vi "1A_Get User Input Start.vi"(1 "Serial Number In":string) -> (0 "fXpgIdentity Output":T1)   [LabVIEW 2010]
panel:
  in  "Stellar \"QIG\" Serial Number":string
  in  "Continue Button":bool
  in  "Device SERIAL Number":string
  in  "PCB LOT Number":string
  # "Enter All Device Parameters Below.\nWhen finished, click \"Continue\"."
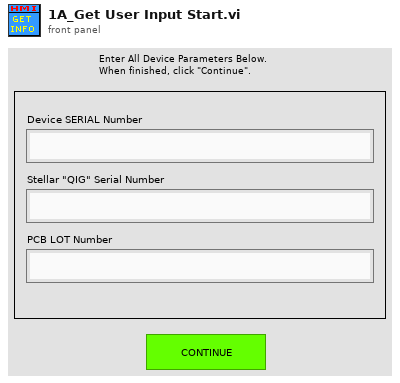
[diagram p1: front panel]
types:
  T1 = cluster{"xpgPCBLotNumber":string, "xpgSerialNumber[20]":string, "xpgStellarQIGSerialNumber":string}
  T2 = cluster{"xpgPCBLOTNumber":string, "xpgSerialNumber[20]":string, "xpgStellarQIGSerialNumber":string}
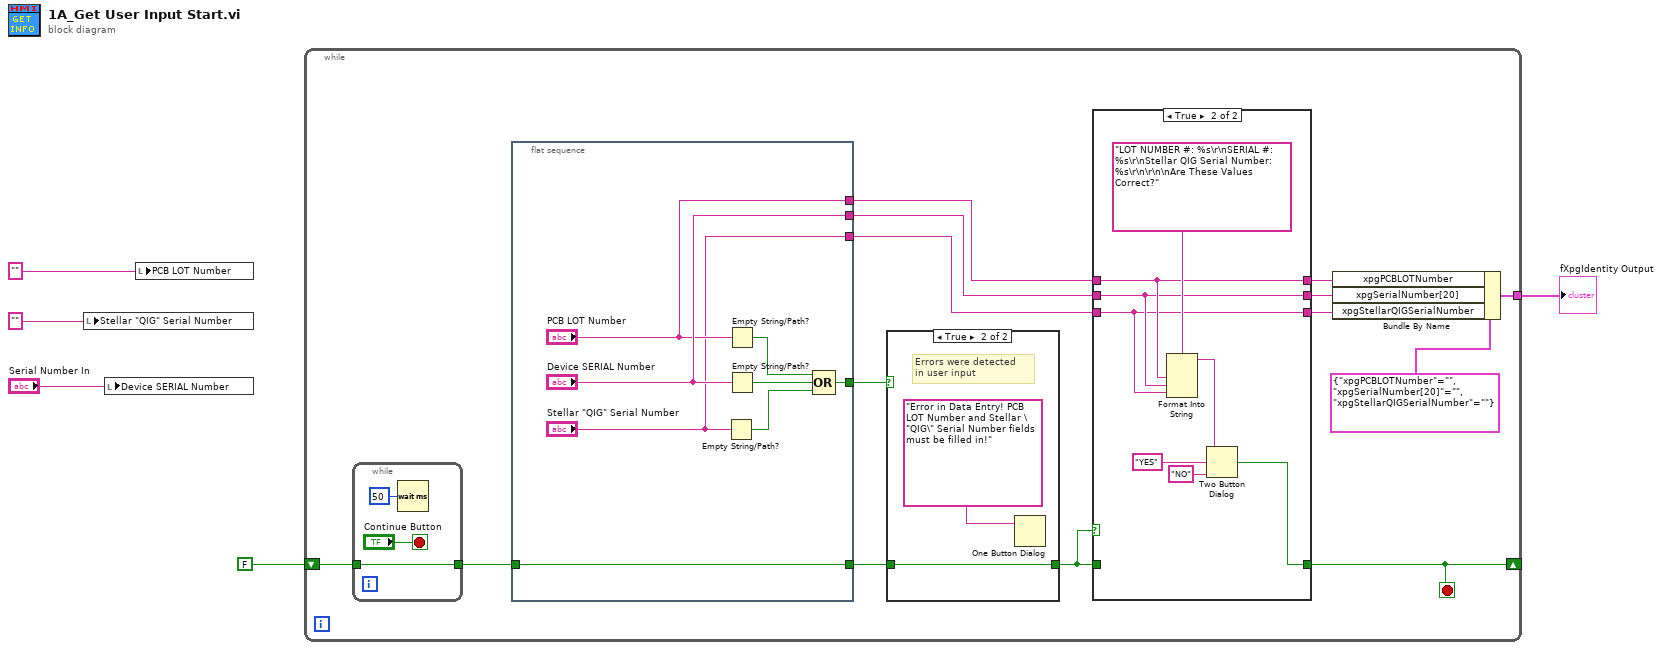
[diagram p0: block diagram]
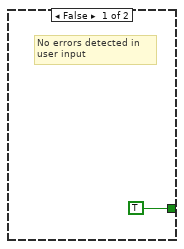
[diagram p3: hidden frame]
diagram:
  n1 = local write "Stellar \"QIG\" Serial Number"("" ("Device LOT Number")) -> ()
  n2 = local write "Device SERIAL Number"("Serial Number In") -> ()
  n3 = local write "PCB LOT Number"("" ("Device LOT Number")) -> ()
  n4 = while {
    shift-right: [w12] -> _
    shift-left: FALSE -> [w19]
    tunnel: [w10] -> w3
    stop <- w12 stop-if-true
    n5 = while {
      tunnel: w19 -> [w45]
      tunnel: [w45] -> w17
      stop <- "Continue Button" stop-if-true
      n6 = Wait (ms)(milliseconds to wait=u32 50) -> ()  [unwired: 1 out]
    }
    n7 = flat-sequence {
      tunnel: [w37] -> w18
      tunnel: ["Device SERIAL Number"] -> w13
      tunnel: ["PCB LOT Number"] -> w14
      tunnel: w17 -> [w34]
      tunnel: [w34] -> w16
      tunnel: ["Stellar \"QIG\" Serial Number"] -> w9
      frame #0 {
        n8 = Empty String/Path?(string/path="Stellar \"QIG\" Serial Number") -> (empty?=w33:bool)
        n9 = Empty String/Path?(string/path="PCB LOT Number") -> (empty?=w38:bool)
        n10 = Empty String/Path?(string/path="Device SERIAL Number") -> (empty?=w39:bool)
        n11 = Compound Arithmetic op=OR(w38, w39, w33) -> (w37:bool)
      }
    }
    n12 = case shown="True" w18 {
      tunnel: w16 -> [_ w42]
      tunnel: [TRUE w42] -> w15
      frame False {
        # "No errors detected in\nuser input"
      }
      frame True {
        # "Errors were detected\nin user input"
        n13 = One Button Dialog(message="Error in Data Entry! PCB LOT Number and Stellar \"QIG\" Serial Number fields must be filled in!") -> ()  [unwired: 1 in, 1 out]
      }
    }
    n14 = case shown="True" w15 {
      tunnel: w15 -> [w23 _]
      tunnel: w14 -> [w22 w26]
      tunnel: w13 -> [w21 w25]
      tunnel: [w23 w27] -> w12
      tunnel: [w22 w26] -> w8
      tunnel: [w21 w25] -> w7
      tunnel: w9 -> [w20 w24]
      tunnel: [w20 w24] -> w6
      frame False {
      }
      frame True {
        n15 = Format Into String(format string="LOT NUMBER #: %s\r\nSERIAL #: %s\r\nStellar QIG Serial Number: %s\r\n\r\n\nAre These Values Correct?", w26, w25, w24) -> (resulting string=w30:string)  [unwired: 2 in, 1 out]
        n16 = Two Button Dialog(message=w30, 1:"NO" ("F button name (\"Cancel\")"), 2:"YES" ("T button name (\"OK\")")) -> (T button?=w27:bool)
      }
    }
    n17 = Bundle By Name(cluster=T2 {"xpgPCBLOTNumber"="", "xpgSerialNumber[20]"="", "xpgStellarQIGSerialNumber"=""} ("fXpgIdentity Output"), "xpgPCBLOTNumber"=w8, "xpgSerialNumber[20]"=w7, "xpgStellarQIGSerialNumber"=w6) -> (w10:T2)
  }
  "fXpgIdentity Output" <- w3
